vi "Test R_W.vi"() -> ()   [LabVIEW 2021]
uses:
  <vilib>/CIF Foundation/CIF Channels Core/CIFChannels/Typedef/Direction.ctl
  <vilib>/CIF Foundation/CIF Channels Core/CIFChannels/CIFChannels.lvclass
  <vilib>/CIF Foundation/CIF Core/CIFCore/Grpc/CIFCoreWrapper/CIFCoreWrapper.lvlib
  <vilib>/CIF Foundation/CIF Core/CIFCore/Grpc/CIFCoreChannel_client/RPC Messages/cif_channelcore_ConnectSubscriber.ctl
  <vilib>/CIF Foundation/CIF Core/CIFCore/Grpc/CIFCoreChannel_client/CIFCoreChannel_client.lvlib
  <vilib>/CIF Foundation/CIF Channels Core/CIPC_Channels/Double/CIF_CIPC_Chn_Double.lvclass
  <vilib>/CIF Foundation/CIF Channels Core/CIPC_Channels/U64/CIF_CIPC_Chn_U64.lvclass
  Common/Template_Common.lvlib
  <vilib>/CIF Foundation/CIF Core/CIFCore/Class/CIFCorePlugin.lvclass
  Common/Typedef/Channels.ctl
  <vilib>/CIF Foundation/CIF Core/CIFCore/Class/Typedef/Energized States.ctl
  <vilib>/CIF Foundation/CIF Channels Core/ChannelCommon/typedef/New FIFO Instance Response.ctl
  <vilib>/CIF Foundation/CIF Channels Core/ChannelCommon/ChannelCommon.lvlib
  <vilib>/CIF Foundation/CIF Core/Channels/CIFChannelMng/CIFChannelMng.lvclass
  <vilib>/CIF Foundation/CIF Core/CIFCore/Common/Typedef/Plugin State.ctl
  <vilib>/CIF Foundation/CIF Core/CIFCore/Common/CIFCoreCommon.lvlib
  <vilib>/CIF Foundation/CIF Core/CIFCore/Common/Typedef/Timing Stats Base.ctl
  <vilib>/CIF Foundation/CIF Core/CIFCore/Common/Typedef/Timing Statistics.ctl
  <vilib>/CIF Foundation/CIF Core/CIFCore/Common/Typedef/FIFO Statistics.ctl
  <vilib>/CIF Foundation/CIF Core/CIFCore/Common/Typedef/Simple Error.ctl
  <vilib>/CIF Foundation/CIF Core/CIFCore/Common/Typedef/Monitor Doubles.ctl
  <vilib>/CIF Foundation/CIF Core/CIFCore/Common/Typedef/Monitor U64.ctl
  <vilib>/CIF Foundation/CIF Core/CIFCore/Common/Typedef/Monitor I64.ctl
  <vilib>/CIF Foundation/CIF Core/CIFCore/Common/Typedef/gRPC Reported Plugin Status.ctl
panel:
  out "Data 4":u64
  out "error out 4":errorcluster
  out "Node Status":T1 {"Monitor Doubles"."4" format="%#_9g"; "Monitor Doubles"."3" format="%#_9g"; "Monitor Doubles"."2" format="%#_9g"; "Monitor Doubles"."1" format="%#_9g"}
  in  "address":string="192.168.1.160:50051"
  in  "Data 3":dbl
  out "error out 3":errorcluster
  in  "stop":bool
  out "error out":errorcluster
  out "Data 2":dbl
  in  "Data":dbl
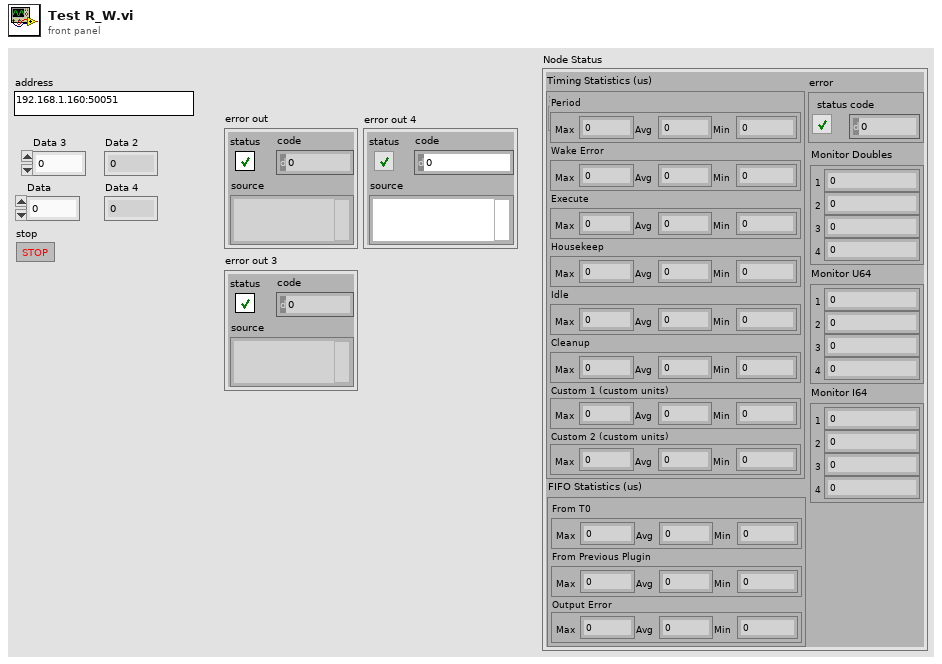
[diagram p1: front panel]
types:
  T1 = typedef "CIFCoreCommon.lvlib/gRPC Reported Plugin Status.ctl" = cluster{"State":T2, "Timing Statistics (us)":T3, "FIFO Statistics (us)":T5, "error":T6, "Monitor Doubles":T7, "Monitor U64":T8, "Monitor I64":T9}
  T2 = typedef "CIFCoreCommon.lvlib/Plugin State.ctl" = enum32{"Null", "Creating", "Listening", "Running", "CleaningUp", "Destroying"}
  T3 = typedef "CIFCoreCommon.lvlib/Timing Statistics.ctl" = cluster{"Period":T4, "Wake Error":T4, "Execute":T4, "Housekeep":T4, "Idle":T4, "Cleanup":T4, "Custom 1 (custom units)":T4, "Custom 2 (custom units)":T4}
  T4 = typedef "CIFCoreCommon.lvlib/Timing Stats Base.ctl" = cluster{"Max":i64, "Avg":dbl, "Min":i64}
  T5 = typedef "CIFCoreCommon.lvlib/FIFO Statistics.ctl" = cluster{"From T0":T4, "From Previous Plugin":T4, "Output Error":T4}
  T6 = typedef "CIFCoreCommon.lvlib/Simple Error.ctl" = cluster{"status":bool, "code":i32}
  T7 = typedef "CIFCoreCommon.lvlib/Monitor Doubles.ctl" = cluster{"1":dbl, "2":dbl, "3":dbl, "4":dbl}
  T8 = typedef "CIFCoreCommon.lvlib/Monitor U64.ctl" = cluster{"1":u64, "2":u64, "3":u64, "4":u64}
  T9 = typedef "CIFCoreCommon.lvlib/Monitor I64.ctl" = cluster{"1":i64, "2":i64, "3":i64, "4":i64}
  T10 = typedef "CIFCoreChannel_client.lvlib/cif_channelcore_ConnectSubscriber.ctl" = cluster{"subscriber_name":string, "publisher_name":string, "custom_connect":u8[]}
  T11 = typedef "CIFChannels.lvclass/Direction.ctl" = enum16{"Publisher", "Subscriber"}
  T12 = typedef "grpc-lvsupport-release.lvlib/grpcId.ctl" = u64
  T13 = typedef "Template_Common.lvlib/Channels.ctl" = enum16{"doubleout", "doublein1", "doublein2", "uint_out", "uint_in", "u8array_out", "u8array_in"}
  T14 = typedef "CIFCorePlugin.lvclass/Energized States.ctl" = enum16{"Listen", "Prepare", "Execute", "Housekeep", "Cleanup", "Destroy"}
  T15 = typedef "ChannelCommon.lvlib/New FIFO Instance Response.ctl" = cluster{"Publisher":string, "Custom Data":u8[]}
  T16 = typedef "ChannelRegistrar.lvlib/Channel Definition.ctl" = cluster{"Name":string, "Direction":T11, "Type":T17, "Custom Config Data":u8[]}
  T17 = typedef "ChannelRegistrar.lvlib/Registered Channel Types.ctl" = enum16{"Custom", "Double_Tag", "I64_Tag", "U64_Tag", "U8_FIFO", "CAN_FIFO", "L2Enet_FIFO", "DAQ_FIFO", "Universal_FIFO", "String_Tag"}
  T18 = typedef "Time_CIF_U.lvlib/Clock Conversion Map.ctl" = map{u8, cluster{"Last Reset":i64, "Offset Pair":T19, "Slope":dbl, "1/Slope":dbl}}
  T19 = typedef "Time_CIF_U.lvlib/Timestamp Pair.ctl" = cluster{"System Time":i64, "External Time":i64}
  T20 = typedef "CIFCoreCommon.lvlib/Channel Connection Data.ctl" = cluster{"Publisher Name":string, "Subscriber Name":string, "Connection Data":u8[]}
  T21 = typedef "CIFCoreCommon.lvlib/Channel Force Data.ctl" = cluster{"Channel Name":string, "Force Data":u8[], "Force Active":bool}
  T22 = typedef "CIFCoreCommon.lvlib/FIFO Publisher.ctl" = cluster{"Publisher Name":string, "New FIFO Instance Config":T23}
  T23 = typedef "ChannelCommon.lvlib/New FIFO Instance Configuration.ctl" = cluster{"Backpressure":bool, "Bytes/Message Override":u32, "Messages/FIFO Override":u32, "Custom Data":u8[]}
  T24 = typedef "CIFChannelMng.lvclass/FIFO Publisher Return.ctl" = cluster{"FIFO Instance Config":T15, "error":errorcluster, "Added":bool}
  T25 = typedef "CIFCoreChannel_client.lvlib/cif_channelcore_Channel.ctl" = cluster{"name":string, "direction":T26, "type":string, "custom_config":u8[], "connected":bool, "connected_name":string, "forced":bool, "channel_pattern":T27}
  T26 = typedef "CIFCoreChannel_client.lvlib/cif_channelcore_Direction.ctl" = enum32{"PUBLISHER", "SUBSCRIBER"}
  T27 = typedef "CIFCoreChannel_client.lvlib/cif_channelcore_PATTERN.ctl" = enum32{"UNKNOWN", "TAG", "FIFO", "MULTIFIFO", "BACKPRESSUREFIFO"}
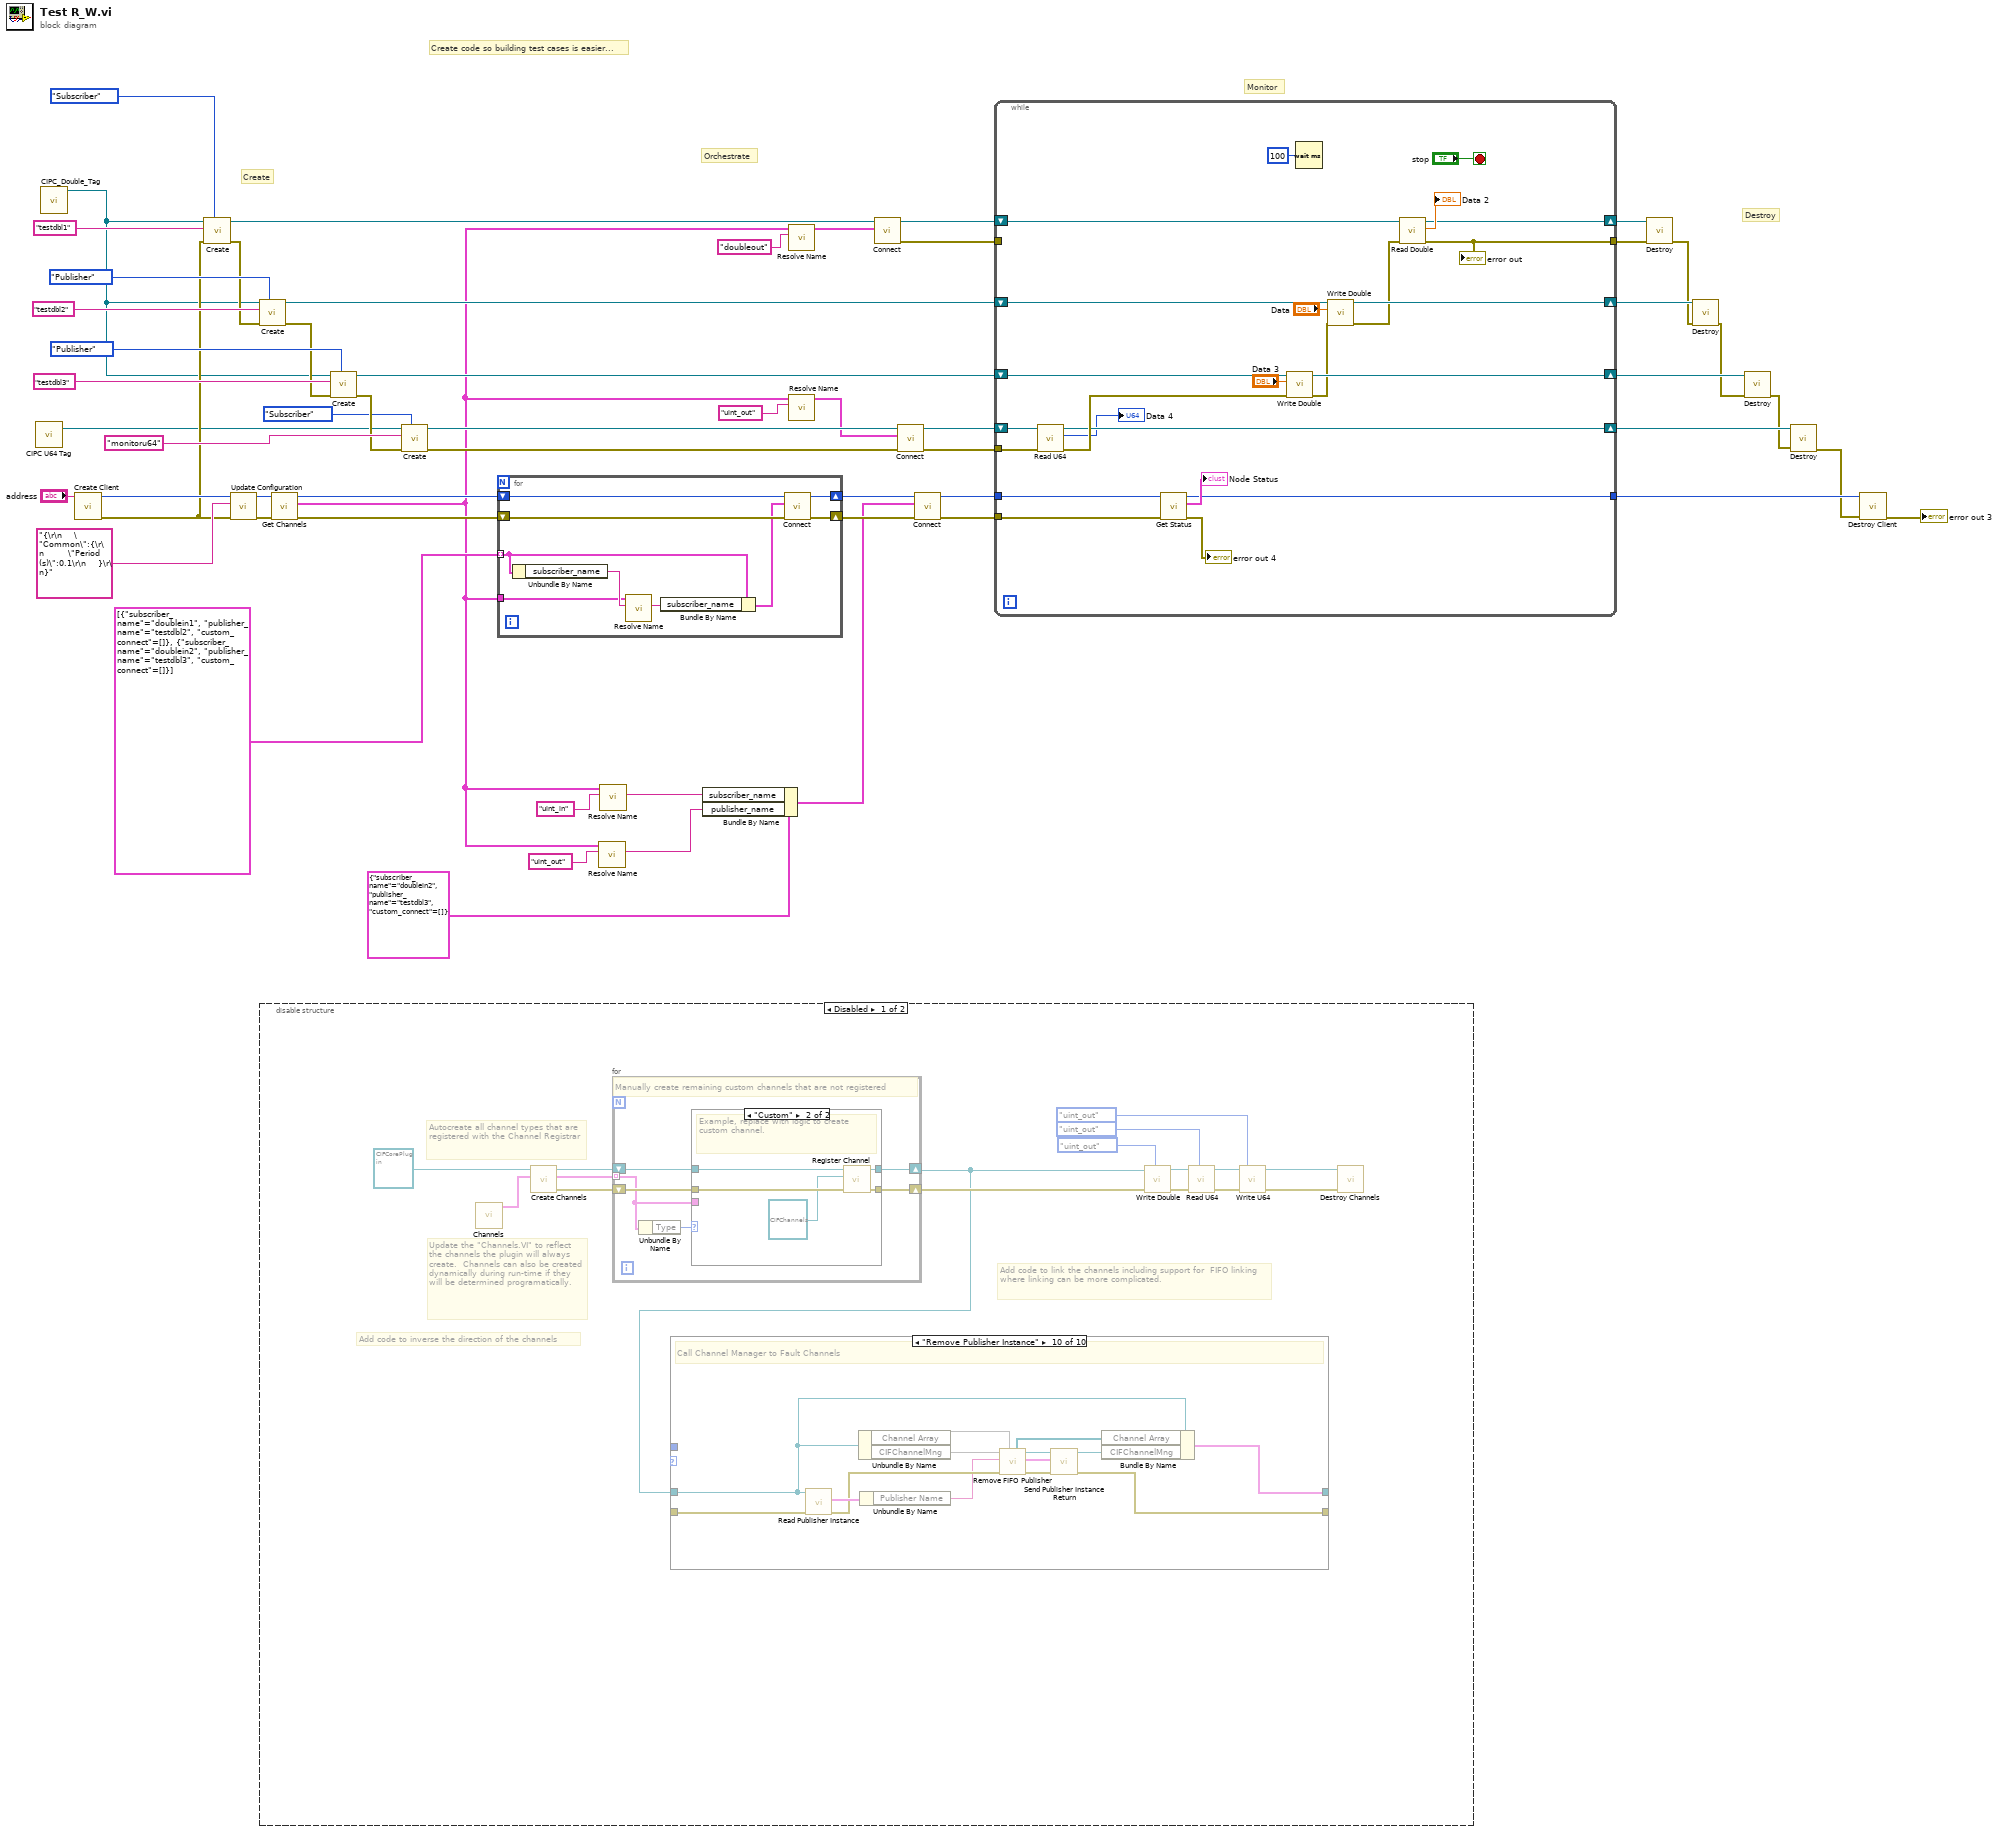
[diagram p0: block diagram]
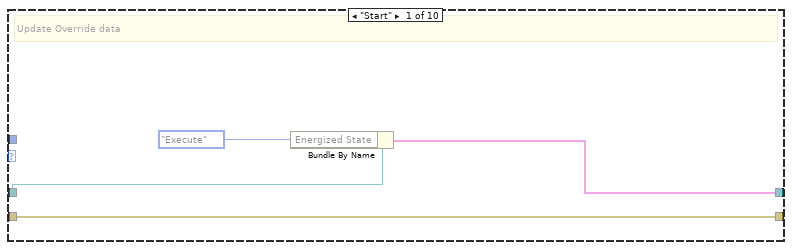
[diagram p2: hidden frame]
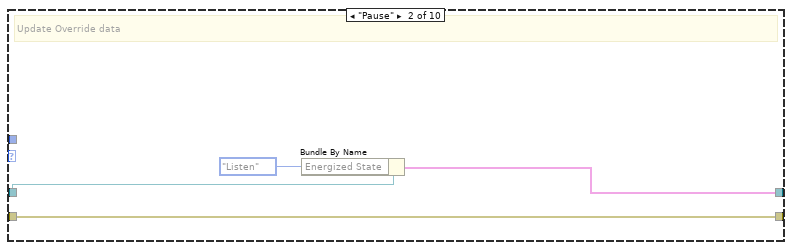
[diagram p3: hidden frame]
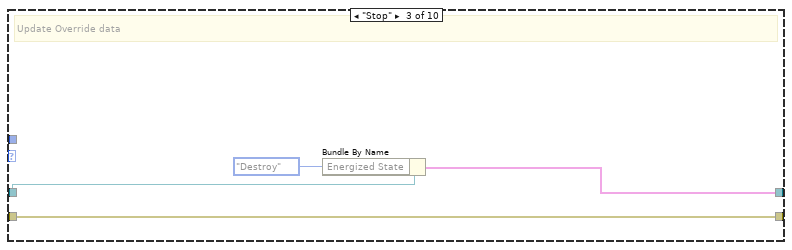
[diagram p4: hidden frame]
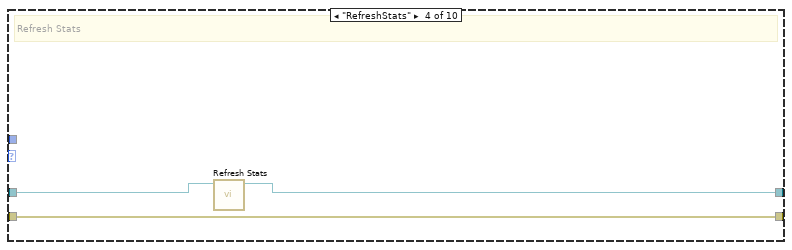
[diagram p5: hidden frame]
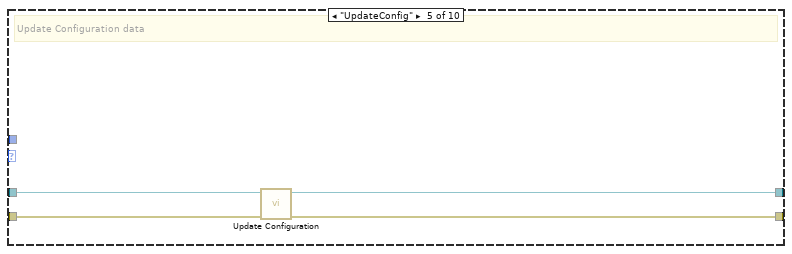
[diagram p6: hidden frame]
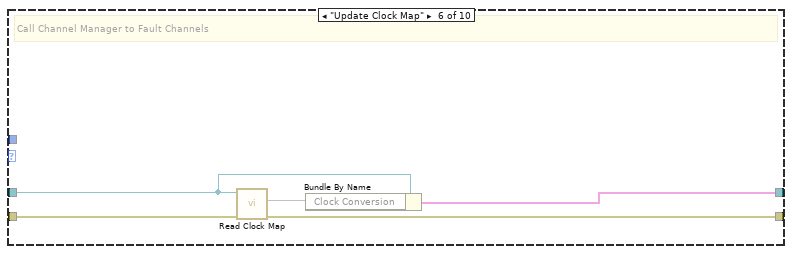
[diagram p7: hidden frame]
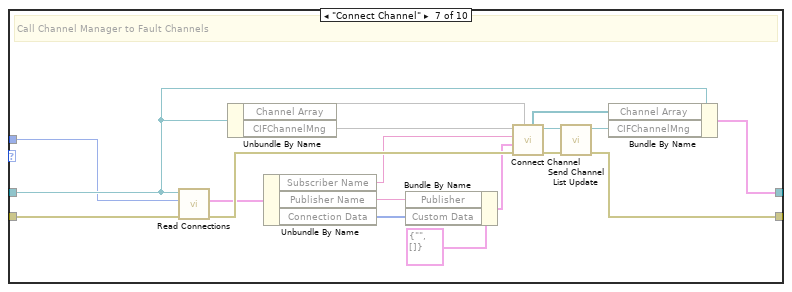
[diagram p8: hidden frame]
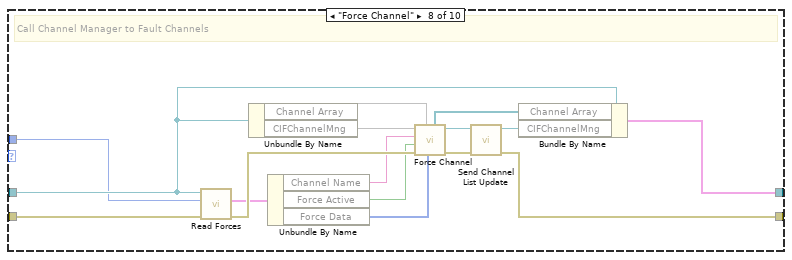
[diagram p9: hidden frame]
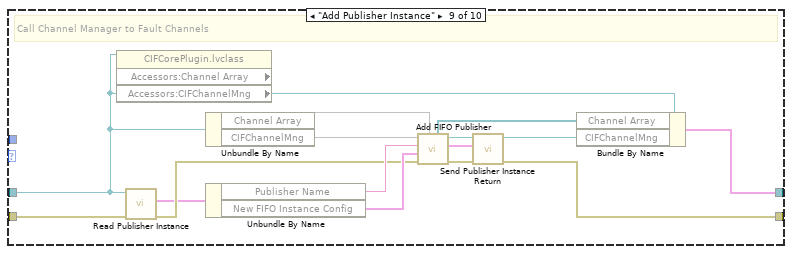
[diagram p10: hidden frame]
diagram:
  # "Create code so building test cases is easier..."
  # "Destroy"
  # "Monitor"
  # "Orchestrate"
  # "Create"
  n1 = call <vilib>:"CIPC U64 Tag.vi"() -> ("CIF_CIPC_Chn_U64.lvclass"=w2:refnum<class "CIF_CIPC_Chn_U64.lvclass">)  [unwired: 11 in]
  n2 = call <vilib>:"CIPC_Double_Tag.vi"() -> ("CIF_CIPC_Chn_Double.lvclass"=w1:refnum<class "CIF_CIPC_Chn_Double.lvclass">)  [unwired: 11 in]
  n3 = call <vilib>:"Create Client.vi"("address"="address") -> ("error out"=w24:errorcluster, "gRPC ID Out"=w25:T12)  [unwired: 9 in]
  n4 = call-dynamic "Create.vi"("Direction"=Direction."Subscriber", "error in (no error)"=w24, "Name"="testdbl1", "CIFTag in"=w1) -> ("error out"=w52:errorcluster, "CIFTag out"=w39:refnum<class "CIF_CIPC_Chn_Double.lvclass">)  [unwired: 6 in]
  n5 = call <vilib>:"Update Configuration.vi"("error in"=w24, "JSON Configuration"="{\r\n    \"Common\":{\r\n        \"Period (s)\":0.1\r\n    }\r\n}" ("JSON Configuration in"), "gRPC ID"=w25) -> ("error out"=w22:errorcluster, "gRPC ID out"=w23:T12)  [unwired: 7 in]
  n6 = call-dynamic "Create.vi"("Direction"=Direction."Publisher", "error in (no error)"=w52, "Name"="testdbl2", "CIFTag in"=w1) -> ("error out"=w43:errorcluster, "CIFTag out"=w55:refnum<class "CIF_CIPC_Chn_Double.lvclass">)  [unwired: 6 in]
  n7 = disable-structure shown="Disabled" {
    frame Disabled {
      # "Add code to link the channels including support for  FIFO linking where linking can be more complicated."
      # "Add code to inverse the direction of the channels"
      # "Update the \"Channels.VI\" to reflect the channels the plugin will always create.  Channels can also be created dynamically during run-time if they will be determined programatically."
      # "Autocreate all channel types that are registered with the Channel Registrar"
      n8 = call "Channels.vi"() -> ("Channels to Create"=w73:T16[])  [unwired: 10 in, 1 out]
      n9 = call <vilib>:"Create Channels.vi"("Channels to Create in"=w73, "CIFCorePlugin in"=refnum<class "CIFCorePlugin.lvclass"> refnum) -> ("error out"=w70:errorcluster, "Channels to Create out"=w72:T16[], "CIFCorePlugin out"=w71:refnum<class "CIFCorePlugin.lvclass">)  [unwired: 7 in]
      n10 = for {
        tunnel: w72 -> [w161] mode=indexing
        shift-right: [w164] -> w58
        shift-left: w71 -> [w166]
        shift-right: [w163] -> w69
        shift-left: w70 -> [w165]
        # "Manually create remaining custom channels that are not registered"
        n11 = Unbundle By Name(w161) -> ("Type"=w162:T17)
        n12 = case shown="\"Custom\"" w162 {
          tunnel: w166 -> [w168 w173]
          tunnel: w165 -> [w167 w172]
          tunnel: [w168 w171] -> w164
          tunnel: [w167 w170] -> w163
          tunnel: w161 -> [_ _]
          frame Default {
          }
          frame "Custom" {
            # "Example, replace with logic to create custom channel."
            n13 = call <vilib>:"Register Channel.vi"("error in (no error)"=w172, "Channel"=refnum<class "CIFChannels.lvclass"> refnum, "CIFCorePlugin in"=w173) -> ("error out"=w170:errorcluster, "CIFCorePlugin out"=w171:refnum<class "CIFCorePlugin.lvclass">)  [unwired: 7 in]
          }
        }
      }
      n14 = case shown="\"Remove Publisher Instance\"" {
        selector: _ -> [_ _ _ _ _ _ _ _ _ _]
        tunnel: _ -> [w74 w81 w85 w86 w91 w97 w114 w129 w143 w160]
        tunnel: w58 -> [w75 w80 w84 w88 w92 w93 w106 w118 w132 w147]
        tunnel: [w77 w79 w83 w87 w90 w96 w103 w117 w133 w148] -> _
        tunnel: [w74 w81 w85 w86 w89 w95 w109 w130 w134 w157] -> _
        tunnel: _ -> [_ _ _ _ _ _ w102 w116 _ _]
        frame "Start" {
          # "Update Override data"
          n15 = Bundle By Name(cluster=w75, "Energized State"=Energized_States."Execute" ("Energized States in")) -> (w77:cluster{})
        }
        frame "Pause" {
          # "Update Override data"
          n16 = Bundle By Name(cluster=w80, "Energized State"=Energized_States."Listen" ("Energized States in")) -> (w79:cluster{})
        }
        frame "Stop" {
          # "Update Override data"
          n17 = Bundle By Name(cluster=w84, "Energized State"=Energized_States."Destroy" ("Energized States in")) -> (w83:cluster{})
        }
        frame "RefreshStats" {
          # "Refresh Stats"
          n18 = call <vilib>:"Refresh Stats.vi"("CIFCorePlugin in"=w88) -> ("CIFCorePlugin out"=w87:refnum<class "CIFCorePlugin.lvclass">)  [unwired: 10 in]
        }
        frame "UpdateConfig" {
          # "Update Configuration data"
          n19 = call-dynamic <vilib>:"Update Configuration.vi"("error in (no error)"=w91, "CIFTemplateNode in"=w92) -> ("error out"=w89:errorcluster, "CIFTemplateNode out"=w90:refnum<class "CIFCorePlugin.lvclass">)  [unwired: 8 in]
        }
        frame "Update Clock Map" {
          # "Call Channel Manager to Fault Channels"
          n20 = call <vilib>:"Read Clock Map.vi"("error in"=w97, "CIFCorePlugin in"=w93) -> ("error out"=w95:errorcluster, "Clock Conversion"=w94:T18)  [unwired: 7 in, 1 out]
          n21 = Bundle By Name(cluster=w93, "Clock Conversion"=w94) -> (w96:cluster{})
        }
        frame "Connect Channel" {
          # "Call Channel Manager to Fault Channels"
          n22 = call <vilib>:"Read Connections.vi"("error in"=w114, "index"=w102, "CIFCorePlugin in"=w106) -> ("error out"=w110:errorcluster, "Connection"=w104:T20)  [unwired: 6 in, 1 out]
          n23 = Unbundle By Name(w106) -> ("Channel Array"=w108, "CIFChannelMng"=w115)
          n24 = Unbundle By Name(w104) -> ("Subscriber Name"=w105:string, "Publisher Name"=w100:string, "Connection Data"=w99:u8[])
          n25 = Bundle By Name(cluster=T15 {"Publisher"="", "Custom Data"=[]} ("Connection"), "Publisher"=w100, "Custom Data"=w99) -> (w98:T15)
          n26 = call <vilib>:"Connect Channel.vi"("Channel Array in"=w108, "error in (no error)"=w110, "Connection"=w98, "Subscriber Name"=w105, "CIFChannelMng in"=w115) -> ("error out"=w112:errorcluster, "CIFChannelMng out"=w113:refnum<class "CIFChannelMng.lvclass">, "Channel Array out"=w107:refnum<class "CIFChannels.lvclass">[])  [unwired: 3 in, 1 out]
          n27 = call <vilib>:"Send Channel List Update.vi"("error in (no error)"=w112, "CIFChannelMng in"=w113) -> ("error out"=w109:errorcluster, "CIFChannelMng out"=w111:refnum<class "CIFChannelMng.lvclass">)  [unwired: 8 in]
          n28 = Bundle By Name(cluster=w106, "Channel Array"=w107, "CIFChannelMng"=w111) -> (w103:cluster{})
        }
        frame "Force Channel" {
          # "Call Channel Manager to Fault Channels"
          n29 = call <vilib>:"Read Forces.vi"("error in"=w129, "index"=w116, "CIFCorePlugin in"=w118) -> ("error out"=w127:errorcluster, "Force"=w119:T21)  [unwired: 6 in, 1 out]
          n30 = Unbundle By Name(w118) -> ("Channel Array"=w124, "CIFChannelMng"=w128)
          n31 = Unbundle By Name(w119) -> ("Channel Name"=w122:string, "Force Active"=w121:bool, "Force Data"=w120:u8[])
          n32 = call <vilib>:"Force Channel.vi"("Force Data"=w120, "Channel Array in"=w124, "error in (no error)"=w127, "Force Active"=w121, "Channel Name"=w122, "CIFChannelMng in"=w128) -> ("error out"=w126:errorcluster, "CIFChannelMng out"=w125:refnum<class "CIFChannelMng.lvclass">, "Channel Array out"=w123:refnum<class "CIFChannels.lvclass">[])  [unwired: 2 in, 1 out]
          n33 = call <vilib>:"Send Channel List Update.vi"("error in (no error)"=w126, "CIFChannelMng in"=w125) -> ("error out"=w130:errorcluster, "CIFChannelMng out"=w131:refnum<class "CIFChannelMng.lvclass">)  [unwired: 8 in]
          n34 = Bundle By Name(cluster=w118, "Channel Array"=w123, "CIFChannelMng"=w131) -> (w117:cluster{})
        }
        frame "Add Publisher Instance" {
          # "Call Channel Manager to Fault Channels"
          n35 = property class="CIFCorePlugin.lvclass" props=["Accessors:Channel Array", "Accessors:CIFChannelMng"](reference=w132) -> ()  [unwired: 1 in, 4 out]
          n36 = call <vilib>:"Read Publisher Instance.vi"("error in"=w143, "CIFCorePlugin in"=w132) -> ("error out"=w142:errorcluster, "Publisher Instance"=w141:T22)  [unwired: 7 in, 1 out]
          n37 = Unbundle By Name(w132) -> ("Channel Array"=w137, "CIFChannelMng"=w146)
          n38 = Unbundle By Name(w141) -> ("Publisher Name"=w145:string, "New FIFO Instance Config"=w144:T23)
          n39 = call <vilib>:"Add FIFO Publisher.vi"("Channel Array in"=w137, "error in (no error)"=w142, "New FIFO Instance Config"=w144, "Channel Name"=w145, "CIFChannelMng in"=w146) -> ("error out"=w139:errorcluster, "FIFO Publisher"=w138:T24, "CIFChannelMng out"=w140:refnum<class "CIFChannelMng.lvclass">, "Channel Array out"=w136:refnum<class "CIFChannels.lvclass">[])  [unwired: 2 in, 1 out]
          n40 = call <vilib>:"Send Publisher Instance Return.vi"("error in (no error)"=w139, "Publisher Instance"=w138, "CIFChannelMng in"=w140) -> ("error out"=w134:errorcluster, "CIFChannelMng out"=w135:refnum<class "CIFChannelMng.lvclass">)  [unwired: 7 in]
          n41 = Bundle By Name(cluster=w132, "Channel Array"=w136, "CIFChannelMng"=w135) -> (w133:cluster{})
        }
        frame "Remove Publisher Instance" {
          # "Call Channel Manager to Fault Channels"
          n42 = call <vilib>:"Read Publisher Instance.vi"("error in"=w160, "CIFCorePlugin in"=w147) -> ("error out"=w155:errorcluster, "Publisher Instance"=w159:T22)  [unwired: 7 in, 1 out]
          n43 = Unbundle By Name(w147) -> ("Channel Array"=w150, "CIFChannelMng"=w156)
          n44 = Unbundle By Name(w159) -> ("Publisher Name"=w154:string)
          n45 = call <vilib>:"Remove FIFO Publisher.vi"("Channel Array in"=w150, "error in (no error)"=w155, "Channel Name"=w154, "CIFChannelMng in"=w156) -> ("error out"=w153:errorcluster, "FIFO Publisher"=w152:T24, "CIFChannelMng out"=w151:refnum<class "CIFChannelMng.lvclass">, "Channel Array out"=w149:refnum<class "CIFChannels.lvclass">[])  [unwired: 3 in, 1 out]
          n46 = call <vilib>:"Send Publisher Instance Return.vi"("error in (no error)"=w153, "Publisher Instance"=w152, "CIFChannelMng in"=w151) -> ("error out"=w157:errorcluster, "CIFChannelMng out"=w158:refnum<class "CIFChannelMng.lvclass">)  [unwired: 7 in]
          n47 = Bundle By Name(cluster=w147, "Channel Array"=w149, "CIFChannelMng"=w158) -> (w148:cluster{})
        }
      }
      n48 = call <vilib>:"Write Double.vi"("Channel Index"=Channels."uint_out" ("Channels"), "error in (no error)"=w69, "CIFCorePlugin in"=w58) -> ("error out"=w67:errorcluster, "CIFCorePlugin out"=w68:refnum<class "CIFCorePlugin.lvclass">)  [unwired: 7 in]
      n49 = call <vilib>:"Read U64.vi"("Channel Index"=Channels."uint_out" ("Channels"), "error in (no error)"=w67, "CIFCorePlugin in"=w68) -> ("error out"=w65:errorcluster, "CIFCorePlugin out"=w66:refnum<class "CIFCorePlugin.lvclass">)  [unwired: 6 in, 1 out]
      n50 = call <vilib>:"Write U64.vi"("Channel Index"=Channels."uint_out" ("Channels"), "error in (no error)"=w65, "CIFCorePlugin in"=w66) -> ("error out"=w63:errorcluster, "CIFCorePlugin out"=w64:refnum<class "CIFCorePlugin.lvclass">)  [unwired: 7 in]
      n51 = call <vilib>:"Destroy Channels.vi"("error in (no error)"=w63, "CIFCorePlugin in"=w64) -> ()  [unwired: 7 in, 3 out]
    }
    frame Enabled {
    }
  }
  n52 = call <vilib>:"Get Channels.vi"("error in"=w22, "gRPC ID"=w23) -> ("error out"=w21:errorcluster, "Channels"=w10:T25[], "gRPC ID out"=w20:T12)  [unwired: 7 in]
  n53 = call-dynamic "Create.vi"("Direction"=Direction."Publisher", "error in (no error)"=w43, "Name"="testdbl3", "CIFTag in"=w1) -> ("error out"=w34:errorcluster, "CIFTag out"=w45:refnum<class "CIF_CIPC_Chn_Double.lvclass">)  [unwired: 6 in]
  n54 = call-dynamic "Create.vi"("Direction"=Direction."Subscriber", "error in (no error)"=w34, "Name"="monitoru64", "CIFTag in"=w2) -> ("error out"=w31:errorcluster, "CIFTag out"=w33:refnum<class "CIF_CIPC_Chn_U64.lvclass">)  [unwired: 6 in]
  n55 = for {
    tunnel: T10[] [{"subscriber_name"="doublein1", "publisher_name"="testdbl2", "custom_connect"=[]}, {"subscriber_name"="doublein2", "publisher_name"="testdbl3", "custom_connect"=[]}] -> [w177] mode=indexing
    shift-right: [w180] -> w15
    shift-left: w21 -> [w181]
    shift-right: [w179] -> w16
    shift-left: w20 -> [w182]
    tunnel: w10 -> [w176]
    n56 = Unbundle By Name(w177) -> ("subscriber_name"=w178:string)
    n57 = call <vilib>:"Resolve Name.vi"("Name in"=w178, "Channels"=w176) -> ("Name out"=w174:string)  [unwired: 8 in, 1 out]
    n58 = Bundle By Name(cluster=w177, "subscriber_name"=w174) -> (w175:T10)
    n59 = call <vilib>:"Connect.vi"("error in"=w181, "Connection"=w175, "gRPC ID"=w182) -> ("error out"=w180:errorcluster, "gRPC ID out"=w179:T12)  [unwired: 7 in]
  }
  n60 = call <vilib>:"Resolve Name.vi"("Name in"="uint_out" ("Name"), "Channels"=w10) -> ("Name out"=w4:string)  [unwired: 8 in, 1 out]
  n61 = call <vilib>:"Resolve Name.vi"("Name in"="uint_in" ("Name"), "Channels"=w10) -> ("Name out"=w3:string)  [unwired: 8 in, 1 out]
  n62 = Bundle By Name(cluster=T10 {"subscriber_name"="doublein2", "publisher_name"="testdbl3", "custom_connect"=[]} ("Connection"), "subscriber_name"=w3, "publisher_name"=w4) -> (w12:T10)
  n63 = call <vilib>:"Resolve Name.vi"("Name in"="doubleout" ("Connection Name"), "Channels"=w10) -> ("Connection"=w9:T15)  [unwired: 8 in, 1 out]
  n64 = call <vilib>:"Resolve Name.vi"("Name in"="uint_out" ("Connection Name"), "Channels"=w10) -> ("Connection"=w19:T15)  [unwired: 8 in, 1 out]
  n65 = call-dynamic <vilib>:"Connect.vi"("Connection"=w9, "CIFTag in"=w39) -> ("error out"=w11:errorcluster, "CIFTag out"=w38:refnum<class "CIF_CIPC_Chn_Double.lvclass">)  [unwired: 8 in]
  n66 = call-dynamic <vilib>:"Connect.vi"("error in (no error)"=w31, "Connection"=w19, "CIFTag in"=w33) -> ("error out"=w30:errorcluster, "CIFTag out"=w32:refnum<class "CIF_CIPC_Chn_U64.lvclass">)  [unwired: 7 in]
  n67 = call <vilib>:"Connect.vi"("error in"=w15, "Connection"=w12, "gRPC ID"=w16) -> ("error out"=w13:errorcluster, "gRPC ID out"=w14:T12)  [unwired: 7 in]
  n68 = while {
    shift-right: [w203] -> w51
    shift-left: w38 -> [w193]
    shift-right: [w202] -> w50
    shift-left: w55 -> [w206]
    tunnel: [w200] -> w49
    shift-right: [w197] -> w47
    shift-left: w45 -> [w195]
    tunnel: w14 -> [w191]
    tunnel: w13 -> [w190]
    tunnel: [w188] -> w37
    tunnel: w30 -> [w186]
    shift-right: [w184] -> w29
    shift-left: w32 -> [w187]
    tunnel: w11 -> [_]
    stop <- "stop" stop-if-true
    n69 = call-dynamic <vilib>:"Read U64.vi"("error in (no error)"=w186, "CIFTag in"=w187) -> ("error out"=w185:errorcluster, "Data"=→"Data 4":u64, "CIFTag out"=w184:refnum<class "CIF_CIPC_Chn_U64.lvclass">)  [unwired: 6 in, 1 out]
    n70 = call <vilib>:"Get Status.vi"("error in"=w190, "gRPC ID"=w191) -> ("error out"=→"error out 4":errorcluster, "Node Status"=→"Node Status":T1, "gRPC ID out"=w188:T12)  [unwired: 7 in]
    n71 = call-dynamic <vilib>:"Write Double.vi"("error in (no error)"=w185, "Data"="Data 3", "CIFTag in"=w195) -> ("error out"=w194:errorcluster, "CIFTag out"=w197:refnum<class "CIF_CIPC_Chn_Double.lvclass">)  [unwired: 6 in, 1 out]
    n72 = Wait (ms)(milliseconds to wait=u32 100) -> ()  [unwired: 1 out]
    n73 = call-dynamic <vilib>:"Write Double.vi"("error in (no error)"=w194, "Data"="Data", "CIFTag in"=w206) -> ("error out"=w201:errorcluster, "CIFTag out"=w202:refnum<class "CIF_CIPC_Chn_Double.lvclass">)  [unwired: 6 in, 1 out]
    n74 = call-dynamic "Read Double.vi"("error in (no error)"=w201, "CIFTag in"=w193) -> ("error out"=w200:errorcluster, "Data"=→"Data 2":dbl, "CIFTag out"=w203:refnum<class "CIF_CIPC_Chn_Double.lvclass">)  [unwired: 6 in, 1 out]
    "error out" <- w200
  }
  n75 = call-dynamic "Destroy.vi"("error in (no error)"=w49, "CIFTag in"=w51) -> ("error out"=w48:errorcluster)  [unwired: 8 in, 1 out]
  n76 = call-dynamic "Destroy.vi"("error in (no error)"=w48, "CIFTag in"=w50) -> ("error out"=w42:errorcluster)  [unwired: 8 in, 1 out]
  n77 = call-dynamic "Destroy.vi"("error in (no error)"=w42, "CIFTag in"=w47) -> ("error out"=w28:errorcluster)  [unwired: 8 in, 1 out]
  n78 = call-dynamic "Destroy.vi"("error in (no error)"=w28, "CIFTag in"=w29) -> ("error out"=w27:errorcluster)  [unwired: 8 in, 1 out]
  n79 = call <vilib>:"Destroy Client.vi"("error in"=w27, "gRPC ID"=w37) -> ("error out"=→"error out 3":errorcluster)  [unwired: 9 in]
